vi "MatrixUtil_CoerceSize.vi"(9 "Columns":i32, 10 "Rows":i32, 11 "input matrix":T1) -> (3 "output matrix":T1)   [LabVIEW 2019, in "Trajectory_Library.lvlib"]
doc: "Creates a new LINEAR SYSTEM data cluster with the specified values. \n\n\nInputs: \n - XXX -- XXX.\n\nOutputs:\n - XXX -- XXX."
uses:
  Trajectory_Library.lvlib
  <vilib>/Analysis/Matrix/Datatypes/RealMatrix.ctl
  <vilib>/Analysis/Matrix/NI_Matrix.lvlib
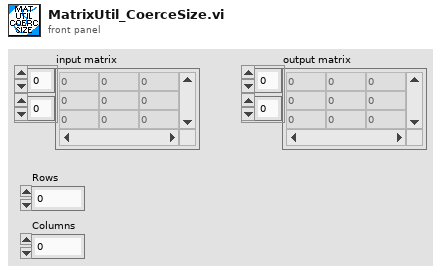
[diagram p1: front panel]
types:
  T1 = typedef "NI_Matrix.lvlib/RealMatrix.ctl" = dbl[][]
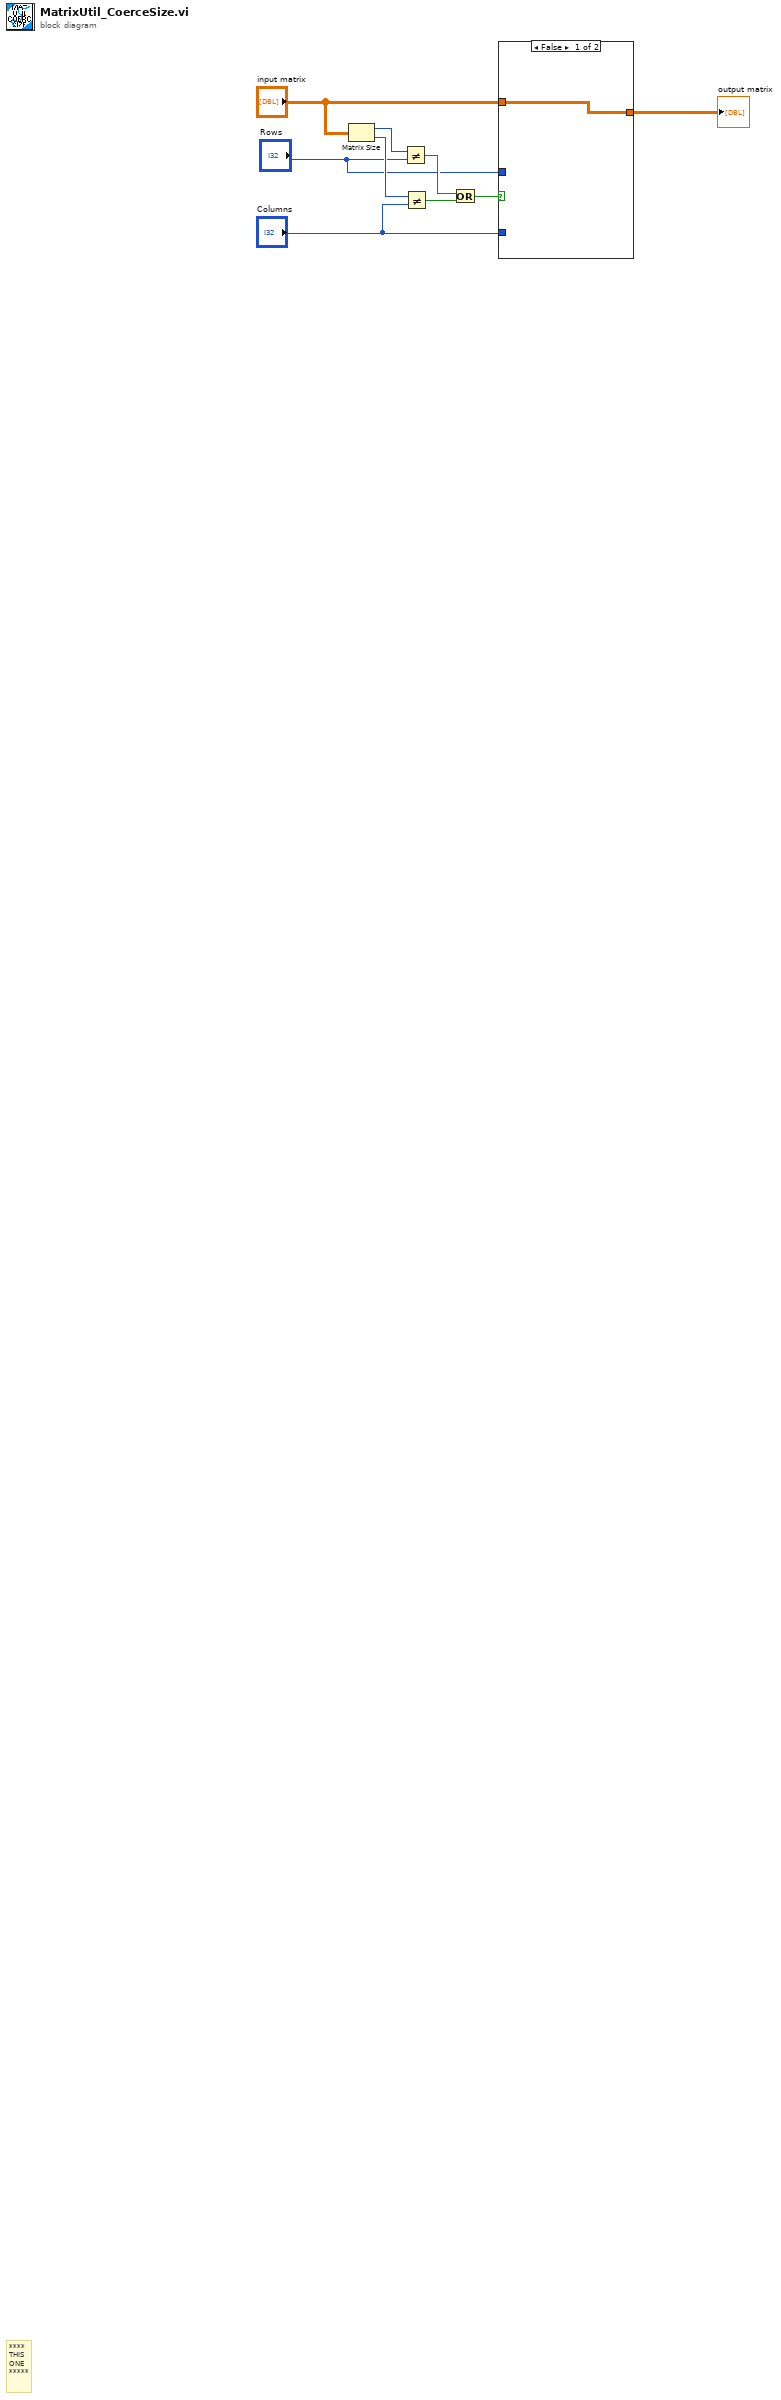
[diagram p0: block diagram]
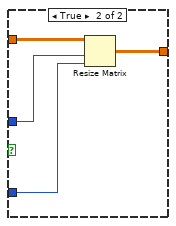
[diagram p2: hidden frame]
diagram:
  # "****\nTHIS\nONE\n*****"
  n1 = Matrix Size(0:"input matrix") -> (1:w7:i32, 2:w8:i32)
  n2 = Not Equal?(x=w7, y="Rows") -> (x != y?=w6:bool)
  n3 = Not Equal?(x=w8, y="Columns") -> (x != y?=w5:bool)
  n4 = Or(x=w6, y=w5) -> (x .or. y?=w9:bool)
  n5 = case shown="False" w9 {
    tunnel: "input matrix" -> [w10 w14]
    tunnel: [w10 w13] -> w3
    tunnel: "Rows" -> [_ w12]
    tunnel: "Columns" -> [_ w11]
    frame False {
    }
    frame True {
      n6 = Resize Matrix(1:w11, 2:w12, 4:w14) -> (0:w13:T1)
    }
  }
  "output matrix" <- w3
